vi "CalculatePSD.vi"(0 "Start Index":i32, 1 "Qfast width":i32=50, 2 "Baseline length":i32=100, 3 "Qtotal width":i32=50, 4 "Chan Wfm":waveform(dbl)) -> (5 "Qfast":dbl, 6 "Qtotal":dbl format="%0.4f")   [LabVIEW 2011]
uses:
  <vilib>/Analysis/2dsp.llb/Integral Method.ctl
  <vilib>/Analysis/8numeric.llb/1D Numeric Integration.vi
  <vilib>/Analysis/NI_AALPro.lvlib
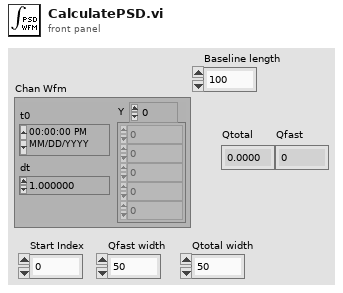
[diagram p1: front panel]
types:
  T1 = typedef "NI_AALPro.lvlib/Integral Method.ctl" = i32
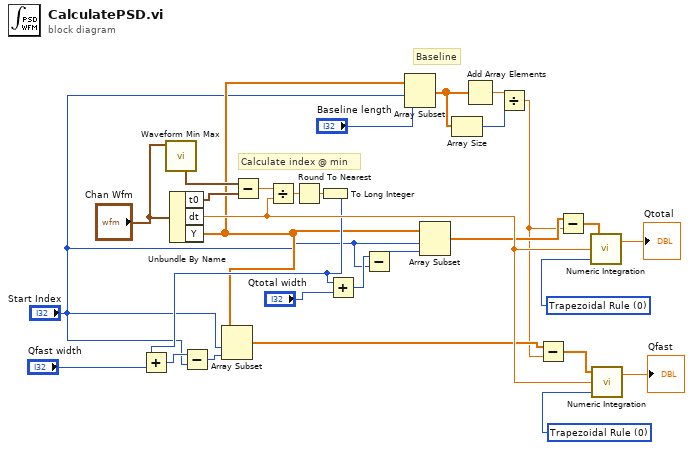
[diagram p0: block diagram]
diagram:
  w27 = T1 0 items=["Trapezoidal Rule", "Simpson's Rule", "Simpson's 3/8 Rule", "Bode Rule"] ("integration method")
  w29 = T1 0 items=["Trapezoidal Rule", "Simpson's Rule", "Simpson's 3/8 Rule", "Bode Rule"] ("integration method")
  # "Baseline"
  # "Calculate index @ min"
  n1 = call <vilib>:"Waveform Min Max.vi"("waveform in"="Chan Wfm") -> ("min time"=w22:timestamp)  [unwired: 5 in, 5 out]
  n2 = Unbundle By Name("Chan Wfm") -> ("t0"=w23:timestamp, "dt"=w20:dbl, "Y"=w11:dbl[])
  n3 = Subtract(x=w22, y=w23) -> (x-y=w21:dbl)
  n4 = Divide(x=w21, y=w20) -> (x/y=w19:dbl)
  n5 = Round To Nearest(number=w19) -> (nearest integer value=w18:dbl)
  n6 = To Long Integer(number=w18) -> (32bit integer=w14:i32)
  n7 = Add(x=w14, y="Qfast width") -> (x+y=w13:i32)
  n8 = Subtract(x=w13, y="Start Index") -> (x-y=w12:i32)
  n9 = Array Subset(array=w11, index="Start Index", length=w12) -> (w4:dbl[])
  n10 = Add(x=w14, y="Qtotal width") -> (x+y=w16:i32)
  n11 = Subtract(x=w16, y="Start Index") -> (x-y=w17:i32)
  n12 = Array Subset(array=w11, index="Start Index", length="Baseline length") -> (w9:dbl[])
  n13 = Array Subset(array=w11, index="Start Index", length=w17) -> (w6:dbl[])
  n14 = Array Size(array=w9) -> (size(s)=w7:i32)
  n15 = Add Array Elements(numeric array=w9) -> (sum=w8:dbl)
  n16 = Divide(x=w8, y=w7) -> (x/y=w3:dbl)
  n17 = Subtract(x=w4, y=w3) -> (x-y=w2:dbl[])
  n18 = Subtract(x=w6, y=w3) -> (x-y=w5:dbl[])
  n19 = call-poly <vilib>:"Numeric Integration.vi"("integration method"=w29, "dt"=w20, "Input Array"=w5) -> ("result"=→"Qtotal":dbl)  [unwired: 1 out]
  n20 = call-poly <vilib>:"Numeric Integration.vi"("integration method"=w27, "dt"=w20, "Input Array"=w2) -> ("result"=→"Qfast":dbl)  [unwired: 1 out]
